vi "helperLoop.vi"(8 "error in (no error)":errorcluster, 11 "Connection Listener in":refnum<class "Connection Listener.lvclass">) -> (0 "error out":errorcluster, 3 "Connection Listener out":refnum<class "Connection Listener.lvclass">)   [LabVIEW 2017, in "Connection Listener.lvlib" / "Connection Listener.lvclass"]
uses:
  Connection Listener.lvclass
  C:/Program Files (x86)/National Instruments/LabVIEW 2017/vi.lib/ActorFramework/Actor/Actor.lvclass
  C:/Users/Public/Documents/wc/BuildFarm/src/LabVIEW/vi.lib/BenjaminR/Build Farm/Actors/Framework/Actor wHelper/Actor wHelper.lvclass
  <vilib>/ActorFramework/Actor/Actor.lvclass/Actor.ctl
  <vilib>/ActorFramework/Message Enqueuer/Message Enqueuer.lvclass/Message Enqueuer.ctl
  Connection Listener.lvclass/Connection Listener.ctl
  Framework/Actor wHelper/Actor wHelper.lvclass/Actor wHelper.ctl
  Connection Listener Messages/New Connection Msg/New Connection Msg.lvclass/New Connection Msg.ctl
  Framework/Actor wHelper/Read StopHelperLoop Reg Ref.vi
  <vilib>/ActorFramework/Message Enqueuer/Init from Existing Queue.vi
  <vilib>/ActorFramework/Message Enqueuer/Enqueue.vi
  Connection Listener Messages/New Connection Msg/New Connection Msg.lvclass
  C:/Program Files (x86)/National Instruments/LabVIEW 2017/vi.lib/ActorFramework/Message/Message.lvclass
  <vilib>/ActorFramework/Stop Msg/Stop Msg.lvclass
  <vilib>/ActorFramework/Message Priority Queue/Priority Enqueue.vi
  <vilib>/ActorFramework/Message Enqueuer/Message Enqueuer.lvclass
  Framework/Actor wHelper/Actor wHelper.lvclass
  <vilib>/MediaMongrels Ltd/WebSockets/Sockets/VISA TCP Listener/VISA TCP Listener.lvclass
  <vilib>/ActorFramework/Actor/Actor.lvclass
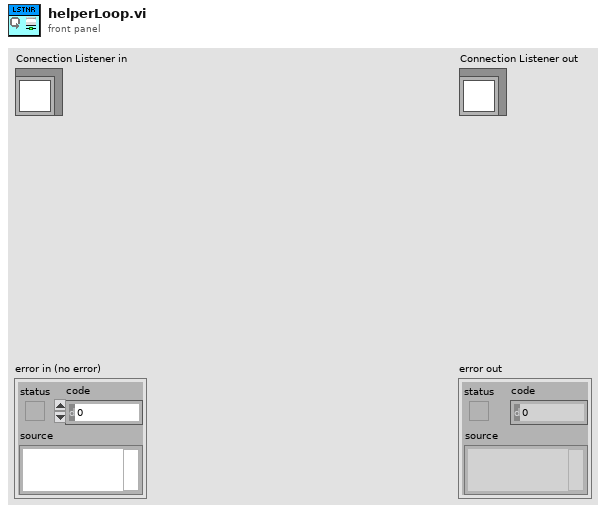
[diagram p1: front panel]
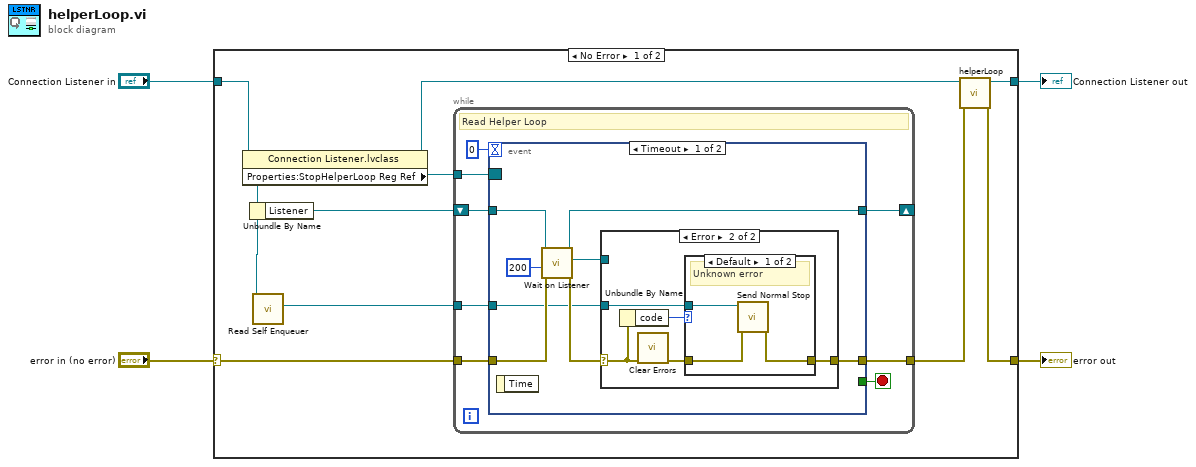
[diagram p0: block diagram]
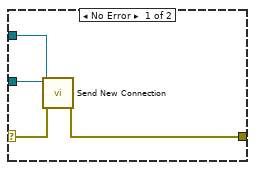
[diagram p2: hidden frame]
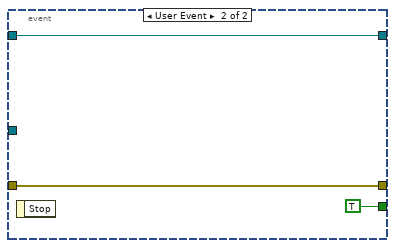
[diagram p4: hidden frame]
diagram:
  n1 = case shown="No Error" "error in (no error)" {
    selector: "error in (no error)" -> [w12 w47]
    tunnel: [w6 w47] -> w2
    tunnel: [w8 w46] -> w3
    tunnel: "Connection Listener in" -> [w5 w46]
    frame No Error {
      n2 = property class="Connection Listener.lvclass"(reference=w5) -> (reference out=w9:refnum<class "Connection Listener.lvclass">, "Properties:StopHelperLoop Reg Ref"=w10:refnum<event-registration>)  [unwired: 1 in, 1 out]
      n3 = Unbundle By Name(w5) -> ("Listener"=w13:refnum<class "VISA TCP Listener.lvclass">)
      n4 = call <vilib>:"Read Self Enqueuer.vi"("Actor"=w5) -> ("Self Enqueuer"=w11:refnum<class "Message Enqueuer.lvclass">)  [unwired: 10 in]
      n5 = while {
        tunnel: w10 -> [w21]
        tunnel: w11 -> [w18]
        shift-right: [w16] -> _
        shift-left: w13 -> [w19]
        tunnel: [w15] -> w7
        tunnel: w12 -> [w14]
        stop <- w20 stop-if-true
        # "Read Helper Loop"
        n6 = event shown="[0] Timeout" {
          selector: w21 -> [_ _]
          dyn-events: _ -> [_ _]
          timeout: 0 -> [_ _]
          tunnel: [_ TRUE] -> w20
          tunnel: w19 -> [w28 w44]
          tunnel: w18 -> [w23 _]
          tunnel: [w22 w44] -> w16
          tunnel: [w29 w43] -> w15
          tunnel: w14 -> [w26 w43]
          event Timeout {
            n7 = event-data() -> ()  [unwired: 1 in, 1 out]
            n8 = call-dynamic "Wait on Listener.vi"("error in (no error)"=w26, "timeout ms (5000)"=200, "VISA TCP Listener in"=w28) -> ("error out"=w25:errorcluster, "Socket out"=w24:refnum<class "Socket.lvclass">, "VISA TCP Listener out"=w22:refnum<class "VISA TCP Listener.lvclass">)  [unwired: 6 in]
            n9 = case shown="Error" w25 {
              selector: w25 -> [w31 w37]
              tunnel: w23 -> [w33 w36]
              tunnel: [w30 w34] -> w29
              tunnel: w24 -> [w32 _]
              frame No Error {
                n10 = call "Send New Connection.vi"("error in (no error)"=w31, "Socket"=w32, "Message Enqueuer in"=w33) -> ("error out"=w30:errorcluster)  [unwired: 7 in, 1 out]
              }
              frame Error {
                n11 = Unbundle By Name(w37) -> ("code"=w38:i32)
                n12 = call <vilib>:"Clear Errors.vi"("error in (no error)"=w37) -> ("error out"=w35:errorcluster)  [unwired: 5 in, 1 out]
                n13 = case shown="Default" w38 {
                  tunnel: w35 -> [w39 w42]
                  tunnel: [w40 w42] -> w34
                  tunnel: w36 -> [w41 _]
                  frame Default {
                    # "Unknown error"
                    n14 = call <vilib>:"Send Normal Stop.vi"("error in (no error)"=w39, "Message Enqueuer"=w41) -> ("error out"=w40:errorcluster)  [unwired: 9 in]
                  }
                  frame 56 {
                    # "Ignore Timeout"
                  }
                }
              }
            }
          }
          event User Event {
            n15 = event-data() -> ()  [unwired: 1 in, 1 out]
          }
        }
      }
      n16 = call-parent "helperLoop.vi"("error in (no error)"=w7, "Actor wHelper in"=w9) -> ("error out"=w6:errorcluster, "Actor wHelper out"=w8:refnum<class "Connection Listener.lvclass">)  [unwired: 8 in]
    }
    frame Error {
    }
  }
  "error out" <- w2
  "Connection Listener out" <- w3
